vi "getOpenPort.vi"() -> (0 "port":u16)   [LabVIEW 2012]
doc: "Returns a local port not currently in use."
uses:
  _ROSDefinition.vi
panel:
  out "Tries":i32
  out "error out":errorcluster
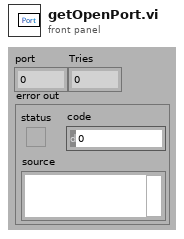
[diagram p1: front panel]
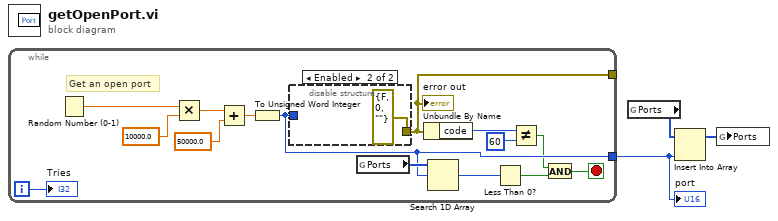
[diagram p0: block diagram]
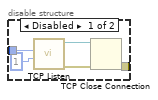
[diagram p2: hidden frame]
diagram:
  n1 = while {
    tunnel: [w10] -> w1
    tunnel: [w5] -> _
    i -> [w4]
    stop <- w7 stop-if-true
    # "Get an open port"
    n2 = Random Number (0-1)() -> (number: 0 to 1=w15:dbl)
    n3 = Multiply(x=w15, y=10000.0) -> (x*y=w14:dbl)
    n4 = Add(x=w14, y=50000.0) -> (x+y=w12:dbl)
    n5 = To Unsigned Word Integer(number=w12) -> (unsigned 16bit integer=w10:u16)
    n6 = disable-structure shown="Enabled" {
      disable-tunnel: w10 -> [w20 _]
      disable-tunnel: [w19 errorcluster {"status"=FALSE, "code"=0, "source"=""} ("error out")] -> w5
      frame Disabled {
        n7 = call <vilib>:"TCP Listen.vi"("timeout ms (wait forever: -1)"=1, "port"=w20) -> ("error out"=w21:errorcluster, "connection ID"=w22:refnum<k5>)  [unwired: 5 in, 3 out]
        n8 = TCP Close Connection(connection ID=w22, error in (no error)=w21) -> (error out=w19:errorcluster)  [unwired: 1 in, 1 out]
      }
      frame Enabled {
      }
    }
    "error out" <- w5
    n9 = global read "_ROSDefinition.vi" "Ports"() -> (w11:u16[])
    n10 = Unbundle By Name(w5) -> ("code"=w18:i32)
    n11 = Search 1D Array(1D array=w11, element=w10) -> (index of element=w9:i32)  [unwired: 1 in]
    n12 = Less Than 0?(x=w9) -> (x < 0?=w8:bool)
    n13 = Not Equal?(x=w18, y=60) -> (x != y?=w6:bool)
    n14 = And(x=w6, y=w8) -> (x .and. y?=w7:bool)
    "Tries" <- w4
  }
  "port" <- w1
  n15 = global read "_ROSDefinition.vi" "Ports"() -> (w3:u16[])
  n16 = Insert Into Array(array=w3, new element=w1) -> (w2:u16[])  [unwired: 1 in]
  n17 = global write "_ROSDefinition.vi" "Ports"(w2) -> ()
